vi "Teleop.vi"(10 "Match Info":T1={"Autonomous Elapsed Seconds"=0.0, "TeleOp Elapsed Seconds"=0.0, "Disabled Elapsed Seconds"=0.0, "Visited Autonomous"=FALSE, "Visited TeleOp"=FALSE, "Visited Disabled"=FALSE, "Autonomous Settings"={"Autonomous Style"=enum."Independent", "VI Refnum"=refnum}}, 11 "Call Context":T2) -> ()   [LabVIEW 2013]
doc: "This VI is called for each TeleOp packet received from the DS where the robot is not disabled. It is often used to read from the joysticks and update I/O or to update setpoints for timed control loops. It should complete and return within 20 milliseconds or it may miss DS packets."
uses:
  <vilib>/Rock Robotics/WPI/DriverStation/WPI_DriverStationDerivedRobotMode.ctl
  <vilib>/Rock Robotics/WPI/DriverStation/WPI_DriverStationMatch Info.ctl
  Robot Global Data.vi
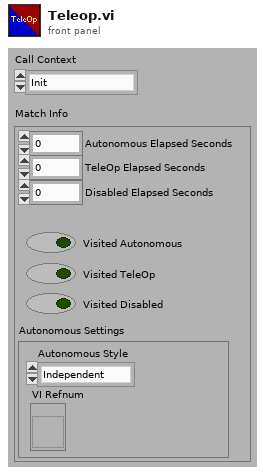
[diagram p1: front panel]
types:
  T1 = typedef "WPI_DriverStationMatch Info.ctl" = cluster{"Autonomous Elapsed Seconds":dbl, "TeleOp Elapsed Seconds":dbl, "Disabled Elapsed Seconds":dbl, "Visited Autonomous":bool, "Visited TeleOp":bool, "Visited Disabled":bool, "Autonomous Settings":cluster{"Autonomous Style":enum16{"Iterative", "Independent"}, "VI Refnum":refnum<vi>}}
  T2 = typedef "WPI_DriverStationDerivedRobotMode.ctl" = enum16{"Init", "Execute", "Stop"}
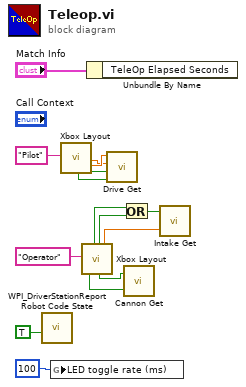
[diagram p0: block diagram]
diagram:
  n1 = call <vilib>:"WPI_DriverStationReport Robot Code State.vi"("TeleOp"=TRUE ("Autonomous")) -> ()  [unwired: 10 in, 1 out]
  n2 = global write "Robot Global Data.vi" "LED toggle rate (ms)"(u32 100 ("LED ms toggle rate")) -> ()
  n3 = call "Xbox Layout.vi"("Joystick Name"="Pilot") -> ("X"=w8:bool, "Right Stick Y"=w10:dbl, "Right Stick X"=w11:dbl, "Right Stick Touch"=w9:bool)  [unwired: 3 in, 12 out]
  n4 = call "Xbox Layout.vi"("Joystick Name"="Operator") -> ("A"=w1:bool, "Left Button"=w3:bool, "Right Button"=w4:bool, "X"=w2:bool, "L+R Throttles"=w6:dbl)  [unwired: 3 in, 11 out]
  n5 = Unbundle By Name("Match Info") -> ()  [unwired: 1 out]
  n6 = call "Drive Get.vi"("Show off spin"=w8, "Slow Drive"=w9, "Y - Axis"=w10, "X - Axis"=w11) -> ()  [unwired: 8 in]
  n7 = Or(x=w3, y=w4) -> (x .or. y?=w5:bool)
  n8 = call "Cannon Get.vi"("Arm?"=w1, "Le Fire At Will?"=w2) -> ()  [unwired: 1 in]
  n9 = call "Intake Get.vi"("Gripper"=w6, "Arm State"=w5) -> ()  [unwired: 1 in]
